vi "BRig_dataLC_Cue_PostR_Count_l2.vi"() -> (2 "output_Cue_PostR_Count_l2":i32)   [LabVIEW 2014]
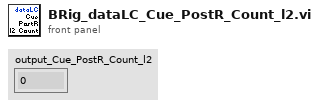
[diagram p1: front panel]
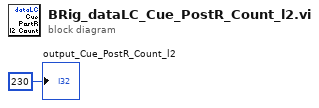
[diagram p0: block diagram]
diagram:
  "output_Cue_PostR_Count_l2" <- 230 ("output_iBlock")
